vi "FormatTableStyle.vi"(7 "Format Command":T1, 8 "Error In":errorcluster, 9 "Row Index":i32, 11 "Table reference Array":refnum<vi>[](array[refnum])) -> (0 "Error Out":errorcluster)   [LabVIEW 2012]
doc: "This VI implements the formatting of table data which includes highlighting, unhighlighting, and modifying visible rows (due to scrolling).\n\n<b>INPUTS</b>\n--------\n<b>Format Command </b> - Formatting action needs to be be taken\n<b>Table references array </b>- Array containing references of the tables of interest\n<b>Row </b>- Row number that needs to be fromatted"
uses:
  FormatTableStyle_Commands.ctl
  <vilib>/Utility/miscctls.llb/LVRowAndColumnTypeDef.ctl
  <vilib>/Utility/miscctls.llb/LVRowAndColumnUnsignedTypeDef.ctl
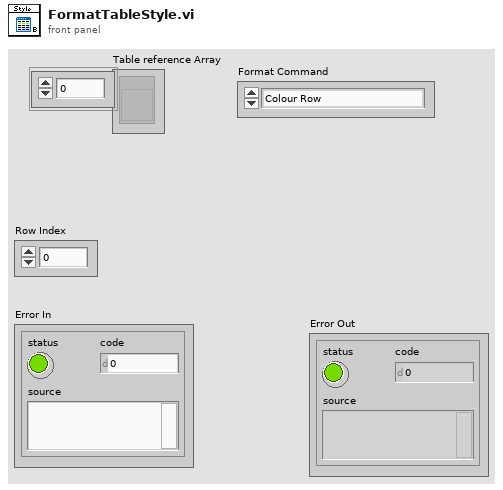
[diagram p1: front panel]
types:
  T1 = typedef "FormatTableStyle_Commands.ctl" = enum16{"Colour Row", "Uncolour Row", "Bold Row", "Clear table", "UpdateVisibleRows"}
  T2 = typedef "LVRowAndColumnTypeDef.ctl" = cluster{"Row":i32, "Column":i32}
  T3 = typedef "LVRowAndColumnUnsignedTypeDef.ctl" = cluster{"Row":u32, "Column":u32}
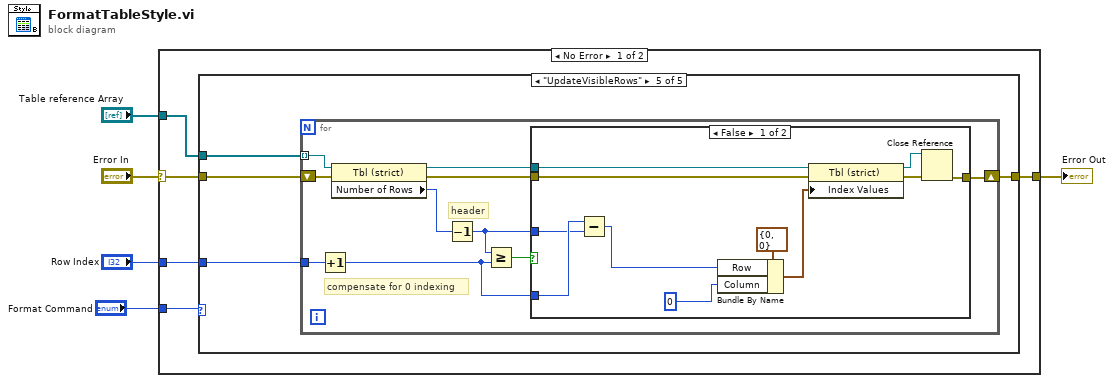
[diagram p0: block diagram]
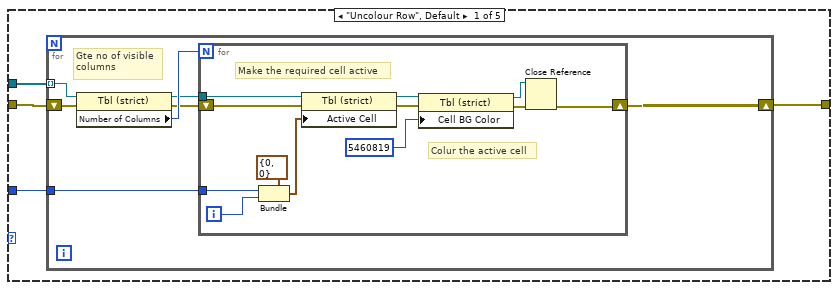
[diagram p2: hidden frame]
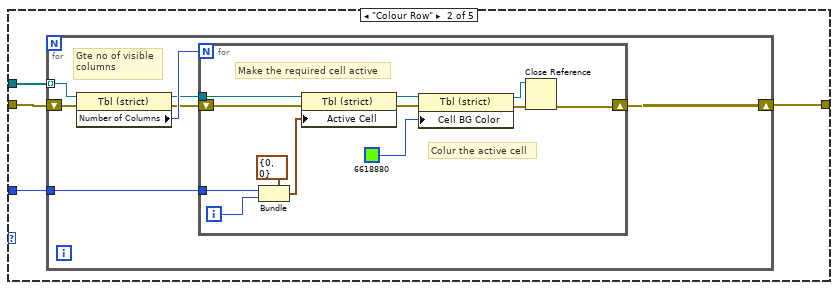
[diagram p3: hidden frame]
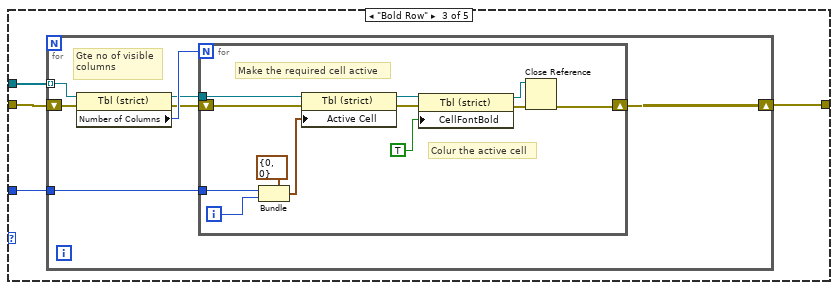
[diagram p4: hidden frame]
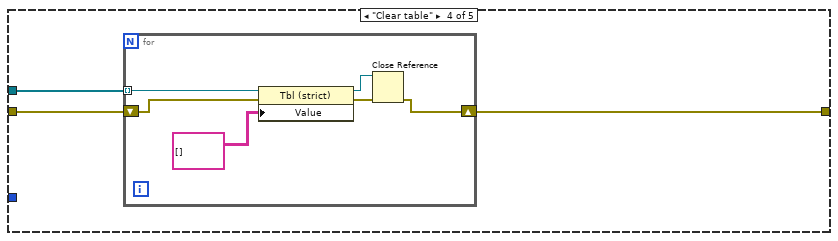
[diagram p5: hidden frame]
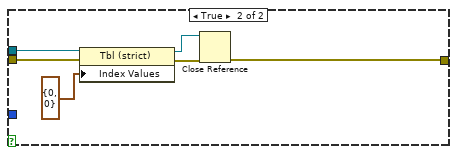
[diagram p6: hidden frame]
diagram:
  n1 = case shown="No Error" "Error In" {
    selector: "Error In" -> [w10 w120]
    tunnel: "Row Index" -> [w8 _]
    tunnel: [w7 w120] -> w3
    tunnel: "Table reference Array" -> [w9 _]
    tunnel: "Format Command" -> [w6 _]
    frame No Error {
      n2 = case shown="\"UpdateVisibleRows\"" w6 {
        tunnel: w10 -> [w14 w37 w60 w80 w91]
        tunnel: w9 -> [w13 w36 w59 w82 w92]
        tunnel: w8 -> [w12 w35 w58 _ w90]
        tunnel: [w11 w34 w57 w81 w89] -> w7
        frame "Uncolour Row", Default {
          n3 = for {
            tunnel: w12 -> [w19]
            tunnel: w13 -> [w21] mode=indexing
            shift-right: [w15] -> w11
            shift-left: w14 -> [w18]
            # "Gte no of visible\ncolumns"
            n4 = property class="Tbl (strict)"(reference=w21, error in=w18) -> (reference out=w17:refnum<vi>, error out=w16:errorcluster, "Number of Columns"=w20:u32)
            n5 = for {
              N: w20 -> [_]
              tunnel: w19 -> [w23]
              tunnel: w17 -> [w29]
              shift-right: [w27] -> w15
              shift-left: w16 -> [w28]
              i -> [w24]
              # "Colur the active cell"
              # "Make the required cell active"
              n6 = Bundle(cluster=T2 {"Row"=0, "Column"=0} ("Active Cell:Active Cell"), "Row"=w23, "Column"=w24) -> (w25:T2)
              n7 = property class="Tbl (strict)"(reference=w29, error in=w28, "Active Cell"=w25) -> (reference out=w33:refnum<vi>, error out=w32:errorcluster)
              n8 = property class="Tbl (strict)"(reference=w33, error in=w32, "Cell BG Color"=u32 5460819 ("Active Cell:Cell Background Color")) -> (reference out=w30:refnum<vi>, error out=w31:errorcluster)
              n9 = Close Reference(reference=w30, error in (no error)=w31) -> (error out=w27:errorcluster)
            }
          }
        }
        frame "Colour Row" {
          n10 = for {
            tunnel: w35 -> [w42]
            tunnel: w36 -> [w44] mode=indexing
            shift-right: [w38] -> w34
            shift-left: w37 -> [w41]
            # "Gte no of visible\ncolumns"
            n11 = property class="Tbl (strict)"(reference=w44, error in=w41) -> (reference out=w40:refnum<vi>, error out=w39:errorcluster, "Number of Columns"=w43:u32)
            n12 = for {
              N: w43 -> [_]
              tunnel: w42 -> [w46]
              tunnel: w40 -> [w52]
              shift-right: [w50] -> w38
              shift-left: w39 -> [w51]
              i -> [w47]
              # "Colur the active cell"
              # "Make the required cell active"
              n13 = Bundle(cluster=T2 {"Row"=0, "Column"=0} ("Active Cell:Active Cell"), "Row"=w46, "Column"=w47) -> (w48:T2)
              n14 = property class="Tbl (strict)"(reference=w52, error in=w51, "Active Cell"=w48) -> (reference out=w56:refnum<vi>, error out=w55:errorcluster)
              n15 = property class="Tbl (strict)"(reference=w56, error in=w55, "Cell BG Color"=u32 6618880 ("Background colour")) -> (reference out=w53:refnum<vi>, error out=w54:errorcluster)
              n16 = Close Reference(reference=w53, error in (no error)=w54) -> (error out=w50:errorcluster)
            }
          }
        }
        frame "Bold Row" {
          n17 = for {
            tunnel: w58 -> [w65]
            tunnel: w59 -> [w67] mode=indexing
            shift-right: [w61] -> w57
            shift-left: w60 -> [w64]
            # "Gte no of visible\ncolumns"
            n18 = property class="Tbl (strict)"(reference=w67, error in=w64) -> (reference out=w63:refnum<vi>, error out=w62:errorcluster, "Number of Columns"=w66:u32)
            n19 = for {
              N: w66 -> [_]
              tunnel: w65 -> [w69]
              tunnel: w63 -> [w75]
              shift-right: [w73] -> w61
              shift-left: w62 -> [w74]
              i -> [w70]
              # "Colur the active cell"
              # "Make the required cell active"
              n20 = Bundle(cluster=T2 {"Row"=0, "Column"=0} ("Active Cell:Active Cell"), "Row"=w69, "Column"=w70) -> (w71:T2)
              n21 = property class="Tbl (strict)"(reference=w75, error in=w74, "Active Cell"=w71) -> (reference out=w79:refnum<vi>, error out=w78:errorcluster)
              n22 = property class="Tbl (strict)"(reference=w79, error in=w78, "CellFontBold"=TRUE ("Active Cell:Cell Font:Bold")) -> (reference out=w76:refnum<vi>, error out=w77:errorcluster)
              n23 = Close Reference(reference=w76, error in (no error)=w77) -> (error out=w73:errorcluster)
            }
          }
        }
        frame "Clear table" {
          n24 = for {
            tunnel: w82 -> [w87] mode=indexing
            shift-right: [w85] -> w81
            shift-left: w80 -> [w83]
            n25 = property class="Tbl (strict)"(reference=w87, error in=w83, "Value"=string[][] []) -> (reference out=w84:refnum<vi>, error out=w88:errorcluster)
            n26 = Close Reference(reference=w84, error in (no error)=w88) -> (error out=w85:errorcluster)
          }
        }
        frame "UpdateVisibleRows" {
          n27 = for {
            tunnel: w92 -> [w102] mode=indexing
            shift-right: [w96] -> w89
            shift-left: w91 -> [w101]
            tunnel: w90 -> [w100]
            # "compensate for 0 indexing"
            # "header"
            n28 = Increment(x=w100) -> (x+1=w95:i32)
            n29 = property class="Tbl (strict)"(reference=w102, error in=w101) -> (reference out=w97:refnum<vi>, error out=w98:errorcluster, "Number of Rows"=w94:u32)
            n30 = Decrement(x=w94) -> (x-1=w93:u32)
            n31 = Greater Or Equal?(x=w93, y=w95) -> (x >= y?=w99:bool)
            n32 = case shown="False" w99 {
              tunnel: w98 -> [w112 w118]
              tunnel: w97 -> [w113 w119]
              tunnel: [w110 w115] -> w96
              tunnel: w93 -> [w104 _]
              tunnel: w95 -> [w105 _]
              frame False {
                n33 = Subtract(x=w105, y=w104) -> (x-y=w103:u32)
                n34 = Bundle By Name(cluster=T3 {"Row"=0, "Column"=0} ("Index Values"), "Row"=w103, "Column"=u32 0) -> (w106:T3)
                n35 = property class="Tbl (strict)"(reference=w113, error in=w112, "Index Values"=w106) -> (reference out=w108:refnum<vi>, error out=w109:errorcluster)
                n36 = Close Reference(reference=w108, error in (no error)=w109) -> (error out=w110:errorcluster)
              }
              frame True {
                n37 = property class="Tbl (strict)"(reference=w119, error in=w118, "Index Values"=T3 {"Row"=0, "Column"=0}) -> (reference out=w114:refnum<vi>, error out=w116:errorcluster)
                n38 = Close Reference(reference=w114, error in (no error)=w116) -> (error out=w115:errorcluster)
              }
            }
          }
        }
      }
    }
    frame Error {
    }
  }
  "Error Out" <- w3
